vi "hidSPD Open Session.vi"(8 "error in (no error)":errorcluster, 11 "Device Info":string[](array[string])) -> (0 "error out":errorcluster, 3 "deviceInfo":string)   [LabVIEW 2018, in "hidSPDLibForLabView.lvlib"]
uses:
  hidSPDLibForLabView.lvlib
  <vilib>/Utility/error.llb/Error Cluster From Error Code.vi
  <vilib>/ErrorRing/Error Ring.xnode
  hidSPD DLL files/libSPD.dll
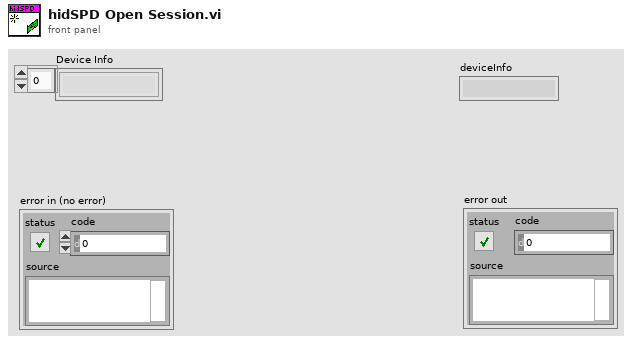
[diagram p1: front panel]
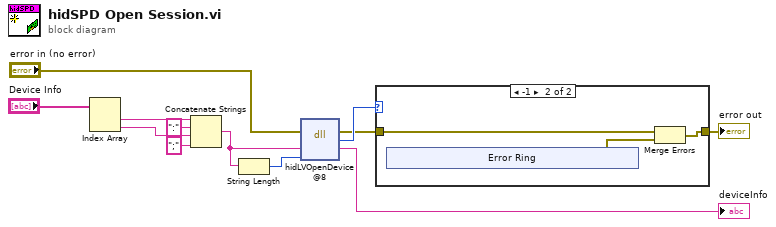
[diagram p0: block diagram]
diagram:
  n1 = Index Array(array="Device Info") -> (element #1=w8:string, element #2=w7:string)  [unwired: 2 in]
  n2 = Concatenate Strings(w8, ":" ("string"), w7, ";" ("string")) -> (w6:string)
  n3 = String Length(string=w6) -> (length=w12:i32)
  n4 = dll-call lib="F:/NextCloud/SPD stand/hidSPDLibForLabView/hidSPD DLL files/libSPD.dll" fn="hidLVOpenDevice@8"(error in="error in (no error)", "deviceInfo"=w6, "infoLength"=w12) -> (error out=w2:errorcluster, "return type"=w4:i32, "deviceInfo"=→"deviceInfo":string)  [unwired: 3 in, 1 out]
  n5 = case shown="-1" w4 {
    tunnel: w2 -> [w13 w16]
    tunnel: [w13 w14] -> w1
    frame 0, Default {
    }
    frame -1 {
      n6 = xnode "Error Ring"() -> ("error out"=w15:errorcluster)
      n7 = Merge Errors(w16, w15) -> (w14:errorcluster)
    }
  }
  "error out" <- w1
